vi "Initialise Actors.vi"(8 "error in (no error)":errorcluster, 11 "Main Controller in":refnum<class "Main Controller Actor.lvclass">) -> (0 "error out":errorcluster, 3 "Main Controller out":refnum<class "Main Controller Actor.lvclass">)   [LabVIEW 2015, in "Main Controller Actor.lvclass"]
uses:
  Main Controller Actor.lvclass
  Re-use Libraries/Minimal Actor Framework/Actors/Base Actor/Actor/Front Panel State.ctl
  Re-use Libraries/Minimal Actor Framework/Actors/Base Actor/Actor/Common Config.ctl
  Re-use Libraries/Minimal Actor Framework/Messaging/Messenger/Messenger.lvclass
  Re-use Libraries/Utility/Get App Paths.vi
  Re-use Libraries/Minimal Actor Framework/Actors/Base Actor/Actor/Actor.lvclass
  Alarm Handler/Actor/Alarm Handler Actor.lvclass
  Task Scheduler/Actor/Task Scheduler Actor.lvclass
  Alarm Handler/API/Alarm Handler Actor API.lvclass
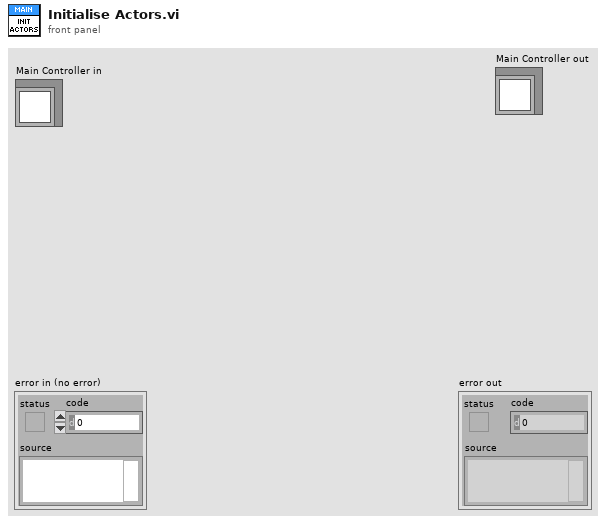
[diagram p1: front panel]
types:
  T1 = typedef "Actor.lvclass/Common Config.ctl" = cluster{"Launch Timeout [ms]":i32, "Wait For Launch Completed":bool, "Front Panel State":T2, "Close FP On Shutdown":bool, "Response Channel":refnum<class "Messenger.lvclass">, "Sub Panel":refnum<vi>}
  T2 = typedef "Actor.lvclass/Front Panel State.ctl" = enum32{"Invalid", "Standard", "Closed", "Hidden", "Minimized", "Maximized"}
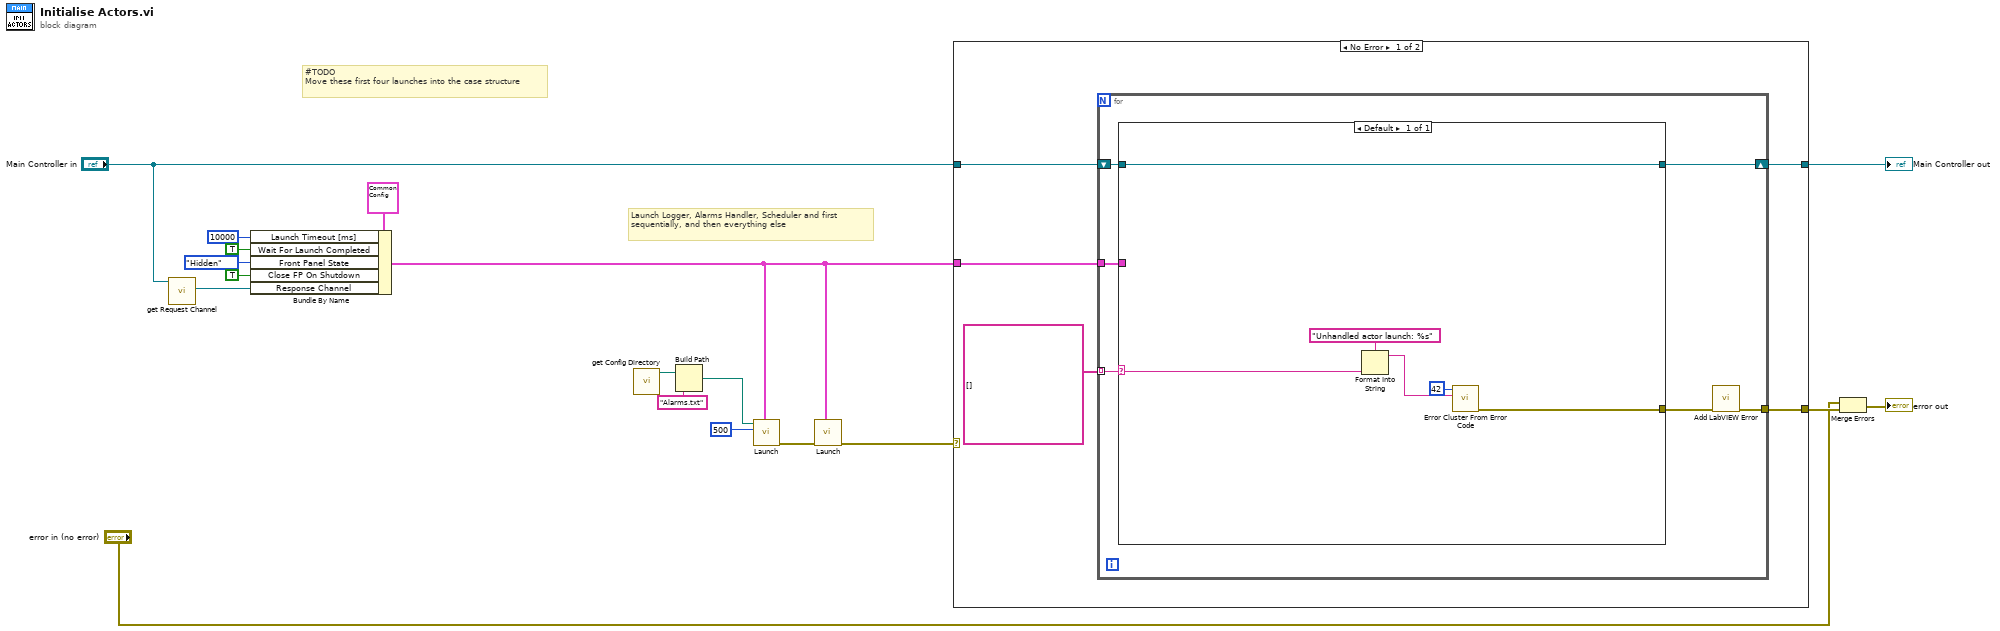
[diagram p0: block diagram]
diagram:
  # "#TODO\nMove these first four launches into the case structure"
  # "Launch Logger, Alarms Handler, Scheduler and first sequentially, and then everything else"
  n1 = call "get Request Channel.vi"("Actor in"="Main Controller in") -> ("Request Channel"=w10:refnum<class "Messenger.lvclass">)  [unwired: 8 in, 2 out]
  n2 = Bundle By Name(cluster=T1 {"Launch Timeout [ms]"=-1, "Wait For Launch Completed"=FALSE, "Front Panel State"=enum."Standard", "Close FP On Shutdown"=TRUE, "Response Channel"=refnum, "Sub Panel"=refnum} ("Config"), "Launch Timeout [ms]"=10000, "Wait For Launch Completed"=TRUE ("Wait For Launch Completed (F)"), "Front Panel State"=Front_Panel_State."Hidden" ("Front Panel State (Standard)"), "Close FP On Shutdown"=TRUE ("Close FP On Shutdown (T)"), "Response Channel"=w10) -> (w4:T1)
  n3 = call "get Config Directory.vi"() -> ("Config Dir"=w6:path)  [unwired: 11 in]
  n4 = Build Path(base path=w6, name or relative path="Alarms.txt") -> (appended path=w5:path)
  n5 = call "Launch.vi"("Common Config"=w4, "Maximum Number Of Errors"=500, "Definitions"=w5) -> ("error out"=w9:errorcluster)  [unwired: 7 in, 1 out]
  n6 = call "Launch.vi"("Common Config"=w4, "error in (no error)"=w9) -> ("error out"=w1:errorcluster)  [unwired: 8 in, 1 out]
  n7 = case shown="No Error" w1 {
    selector: w1 -> [_ w36]
    tunnel: [w19 w36] -> w18
    tunnel: w4 -> [w22 _]
    tunnel: "Main Controller in" -> [w21 w37]
    tunnel: [w20 w37] -> w2
    frame No Error {
      n8 = for {
        tunnel: string[] [] -> [w29] mode=indexing
        tunnel: w22 -> [w28]
        shift-right: [w26] -> w20
        shift-left: w21 -> [w27]
        tunnel: [w24] -> w19
        n9 = case shown="Default" w29 {
          selector: w29 -> [w33]
          tunnel: w28 -> [_]
          tunnel: [w35] -> w25
          tunnel: w27 -> [w30]
          tunnel: [w30] -> w26
          frame Default {
            n10 = Format Into String(format string="Unhandled actor launch: %s", w33) -> (resulting string=w32:string)  [unwired: 2 in, 1 out]
            n11 = call <vilib>:"Error Cluster From Error Code.vi"("error message (\"\")"=w32, "error code (0)"=42) -> ("error out"=w35:errorcluster)  [unwired: 7 in]
          }
        }
        n12 = call "Add LabVIEW Error.vi"("error in (no error)"=w25) -> ("error out"=w24:errorcluster)  [unwired: 10 in]
      }
    }
    frame Error {
    }
  }
  "Main Controller out" <- w2
  n13 = Merge Errors("error in (no error)", w18) -> (→"error out":errorcluster)
